vi "makeMeasSetSelect.vi"(0 "connection reference":refnum<k7>, 2 "meas_setting":T2 {"zStartDistCm" format="%.2f"; "numTxCycles" format="%.1f"; "profTxVoltageVolt" format="%#_1g"; "ceilTxVoltageVolt" format="%.2f"; "maxTxVoltageVolt" format="%.2f"; "focusRangeCm" format="%.1f"; "txFrequencyHz" format="%.2f"}, 3 "condition":string="where", 4 "floating-point type conversion":string[][](table)=[["extended", "5", "12"], ["double", "5", "9"], ["single", "5", "5"]], 5 "error in":T1) -> (6 "connection reference":refnum<k7>, 7 "select sql statement":string, 8 "error out":T1)   [LabVIEW 2016]
doc: "This VI will dynamically create a SELECT SQL statement for meas_setting."
uses:
  type def/measSetting.ctl
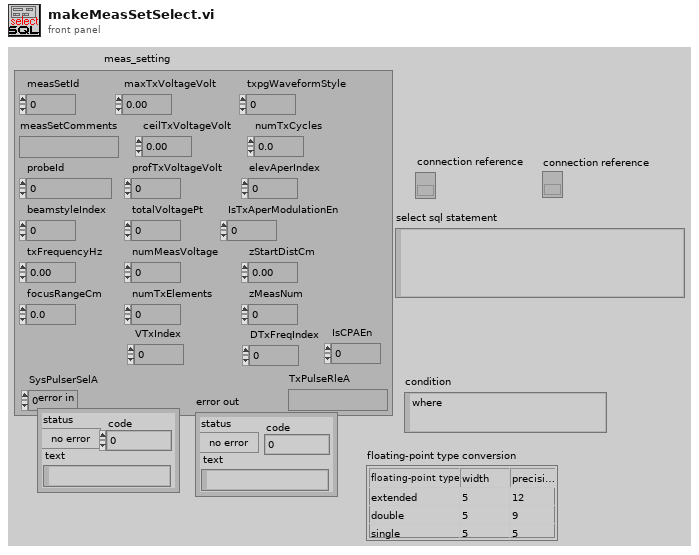
[diagram p1: front panel]
types:
  T1 = cluster{"status":bool, "code":i32, "text":string}
  T2 = typedef "measSetting.ctl" = cluster{"measSetId":i32, "measSetComments":string, "probeId":sgl, "beamstyleIndex":i16, "txFrequencyHz":sgl, "focusRangeCm":sgl, "maxTxVoltageVolt":sgl, "ceilTxVoltageVolt":sgl, "profTxVoltageVolt":dbl, "totalVoltagePt":i8, "numMeasVoltage":i8, "numTxElements":i16, "txpgWaveformStyle":i8, "numTxCycles":sgl, "elevAperIndex":i8, "zStartDistCm":sgl, "zMeasNum":i8, "IsTxAperModulationEn":i8, "DTxFreqIndex":i16, "VTxIndex":i8, "IsCPAEn":i16, "SysPulserSelA":i16, "TxPulseRleA":string}
  T3 = cluster{"name":string, "type  ":u16, "value":string}[]
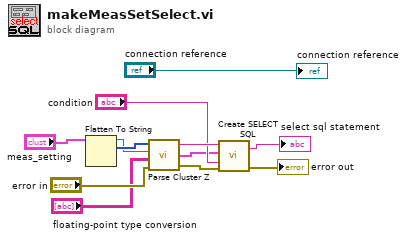
[diagram p0: block diagram]
diagram:
  n1 = Flatten To String(anything="meas_setting") -> (data string=w11:string, type string=w12:i16[])  [unwired: 3 in, 1 out]
  n2 = call "Parse Cluster Z.vi"("error in"="error in", "floating-point type conversion"="floating-point type conversion", "cluster data"=w11, "cluster definition"=w12) -> ("error out"=w7:T1, "cluster controls"=w5:T3, "cluster name"=w8:string)
  n3 = call <vilib>:"Create SELECT SQL.vi"("error in"=w7, "condition"="condition", "column info"=w5, "table name"=w8) -> ("error out"=→"error out":errorcluster, "SQL select statement"=→"select sql statement":string)
  "connection reference" <- "connection reference"
